vi "DeleteSampleInfo.vi"(0 "TCP网络连接输入":refnum<k5>, 5 "Row":dbl, 7 "id":string, 9 "SampleTime":string, 11 "错误输入（无错误）":errorcluster) -> (6 "删除？":bool, 15 "错误输出":errorcluster)   [LabVIEW 2014]
panel:
  out "连接的字符串":string
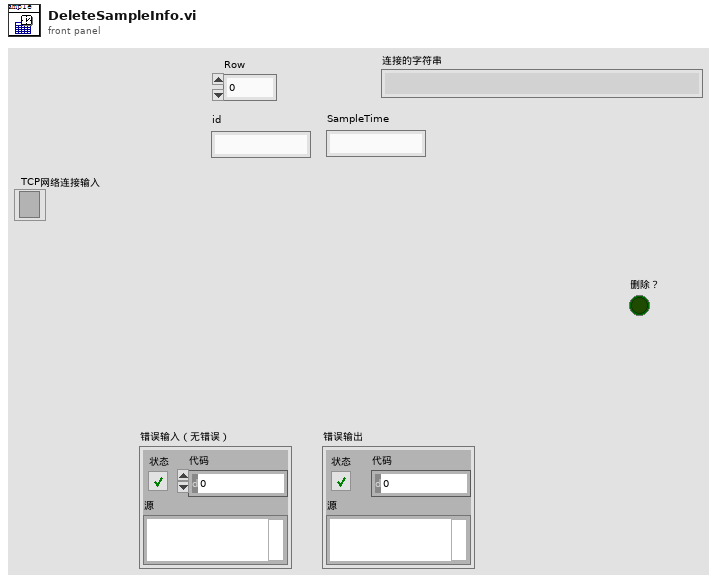
[diagram p1: front panel]
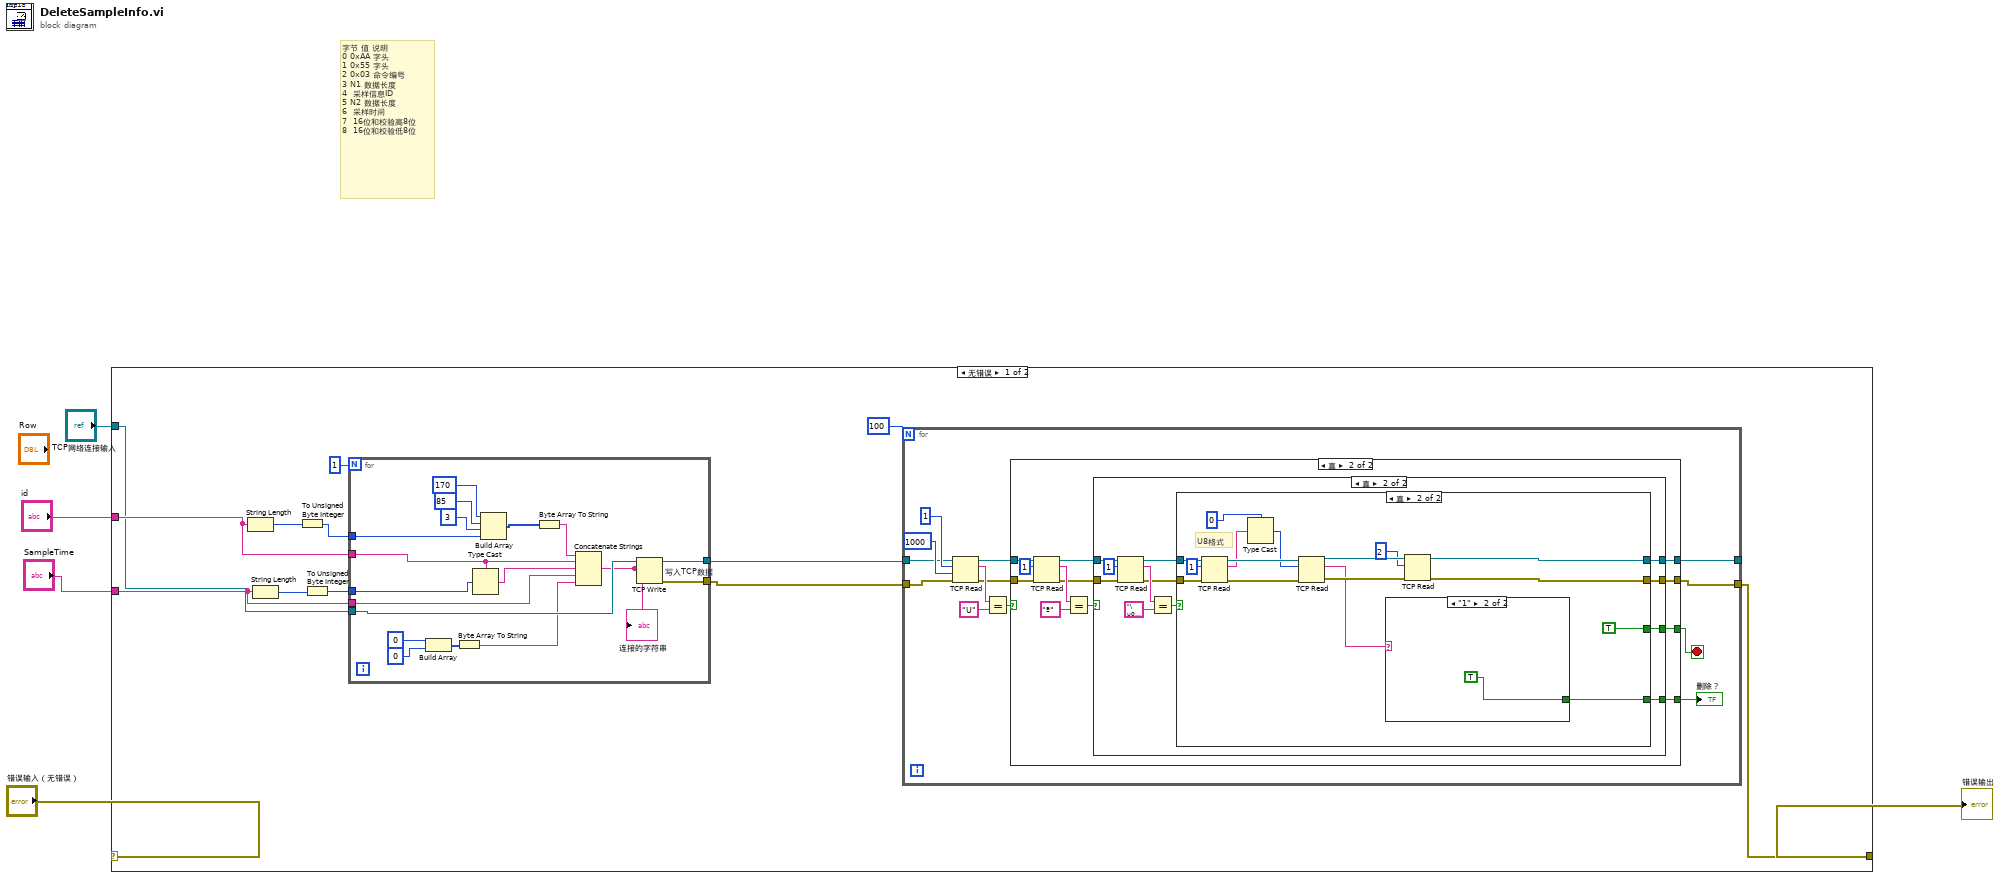
[diagram p0: block diagram]
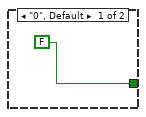
[diagram p5: hidden frame]
diagram:
  # "字节\t值\t说明\n0\t0xAA\t字头\n1\t0x55\t字头\n2\t0x03\t命令编号\n3\tN1\t数据长度\n4\t\t采样信息ID\n5\tN2\t数据长度\n6\t\t采样时间\n7\t\t16位和校验高8位\n8\t\t16位和校验低8位"
  n1 = case shown="无错误" "错误输入（无错误）" {
    selector: "错误输入（无错误）" -> [_ w97]
    tunnel: [w9 w97] -> w5
    tunnel: "TCP网络连接输入" -> [w6 _]
    tunnel: "id" -> [w13 _]
    tunnel: "SampleTime" -> [w10 _]
    frame No Error {
      n2 = String Length(string=w13) -> (length=w15:i32)
      n3 = String Length(string=w10) -> (length=w12:i32)
      n4 = To Unsigned Byte Integer(number=w15) -> (unsigned 8bit integer=w14:u8)
      n5 = To Unsigned Byte Integer(number=w12) -> (unsigned 8bit integer=w11:u8)
      n6 = for {
        N: 1 -> [_]
        tunnel: [w95] -> w8
        tunnel: w6 -> [w94]
        tunnel: [w96] -> w17
        tunnel: w14 -> [w84]
        tunnel: w13 -> [w82]
        tunnel: w11 -> [w83]
        tunnel: w10 -> [w80]
        n7 = Build Array(u8 0, u8 0) -> (w87:u8[])
        n8 = Byte Array To String(unsigned byte array=w87) -> (string=w79:string)
        n9 = Type Cast(type=w82, x=w83) -> (*(type *) &x=w81:string)
        n10 = Build Array(u8 170, u8 85, u8 3, w84) -> (w90:u8[])
        n11 = Byte Array To String(unsigned byte array=w90) -> (string=w86:string)
        n12 = Concatenate Strings(w86, w82, w81, w80, w79) -> (w85:string)
        "连接的字符串" <- w85
        n13 = TCP Write "写入TCP数据"(connection ID=w94, data in=w85) -> (connection ID out=w96:refnum<k5>, error out=w95:errorcluster)  [unwired: 2 in, 1 out]
      }
      n14 = for "For循环" {
        N: 100 -> [_]
        tunnel: w17 -> [w23]
        tunnel: [w21] -> _
        tunnel: w8 -> [w18]
        tunnel: [w20] -> w9
        stop <- w22 stop-if-true
        n15 = TCP Read(connection ID=w23, bytes to read=1 ("读取的字节"), error in (no error)=w18, 9:1000 ("超时毫秒(25000)")) -> (connection ID out=w26:refnum<k5>, data out=w28:string, error out=w25:errorcluster)  [unwired: 1 in]
        n16 = Equal?(x=w28, y="U") -> (x = y?=w27:bool)
        n17 = case shown="真" w27 {
          tunnel: w26 -> [w32 w41]
          tunnel: w25 -> [w31 w40]
          tunnel: [w32 w36] -> w21
          tunnel: [w31 w35] -> w20
          tunnel: [_ w34] -> w22
          tunnel: [_ w33] -> w19
          frame False {
          }
          frame True {
            n18 = TCP Read(connection ID=w41, bytes to read=1 ("读取的字节"), error in (no error)=w40) -> (connection ID out=w38:refnum<k5>, data out=w42:string, error out=w37:errorcluster)  [unwired: 2 in]
            n19 = Equal?(x=w42, y="ª") -> (x = y?=w39:bool)
            n20 = case shown="真" w39 {
              tunnel: w38 -> [w46 w55]
              tunnel: w37 -> [w45 w54]
              tunnel: [w46 w50] -> w36
              tunnel: [w45 w49] -> w35
              tunnel: [_ w48] -> w34
              tunnel: [_ w47] -> w33
              frame False {
              }
              frame True {
                n21 = TCP Read(connection ID=w55, bytes to read=1 ("读取的字节"), error in (no error)=w54) -> (connection ID out=w53:refnum<k5>, data out=w56:string, error out=w52:errorcluster)  [unwired: 2 in]
                n22 = Equal?(x=w56, y="\u0003") -> (x = y?=w51:bool)
                n23 = case shown="真" w51 {
                  tunnel: w53 -> [w60 w75]
                  tunnel: w52 -> [w59 w74]
                  tunnel: [w60 w67] -> w50
                  tunnel: [w59 w68] -> w49
                  tunnel: [_ TRUE] -> w48
                  tunnel: [_ w61] -> w47
                  frame False {
                  }
                  frame True {
                    # "U8格式"
                    n24 = TCP Read(connection ID=w75, bytes to read=1 ("读取的字节"), error in (no error)=w74) -> (connection ID out=w73:refnum<k5>, data out=w65:string, error out=w72:errorcluster)  [unwired: 2 in]
                    n25 = Type Cast(type=u8 0, x=w65) -> (*(type *) &x=w63:u8)
                    n26 = TCP Read(connection ID=w73, bytes to read=w63, error in (no error)=w72) -> (connection ID out=w70:refnum<k5>, data out=w62:string, error out=w69:errorcluster)  [unwired: 2 in]
                    n27 = case shown="\"1\"" w62 {
                      tunnel: [FALSE TRUE] -> w61
                      frame "0", Default {
                      }
                      frame "1" {
                      }
                    }
                    n28 = TCP Read(connection ID=w70, bytes to read=2 ("读取的字节"), error in (no error)=w69) -> (connection ID out=w67:refnum<k5>, error out=w68:errorcluster)  [unwired: 2 in, 1 out]
                  }
                }
              }
            }
          }
        }
        "删除？" <- w19
      }
    }
    frame Error {
    }
  }
  "错误输出" <- w5
